vi "Test and Get Data.vi"(5 "Point #":i32, 6 "Eng Units?":bool, 7 "error in (no error)":errorcluster, 8 "Instrument Info":T1={"Instrument"="Instrument", "ID Test String"="", "Terminator Character"="", "wait (mS)"=0, "Wait For SRQ"=FALSE}, 9 "Command String":string, 10 "VISA Sesson":refnum<visa-resource-name>) -> (0 "Error Out":errorcluster, 1 "Measurement":dbl[](array[numeric]), 2 "String Response":string, 3 "dup VISA session":refnum<visa-resource-name>, 4 "Stop":bool)   [LabVIEW 2019]
doc: "This VI reads tests for presence of an instrument on the GPIB bus for an index <0. It also gets one reading from an instrument. If no reading is obtained a single zero is returned.\nScott Hannahs, <sth@magnet.fsu.edu> NHMFL-FSU, May 2003"
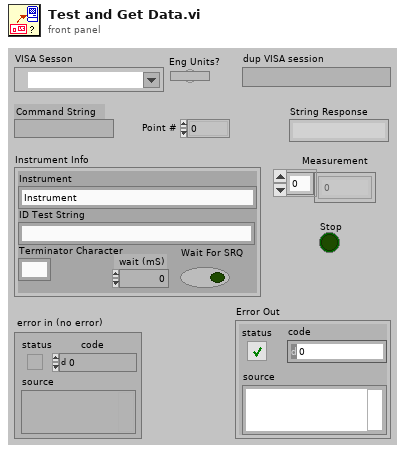
[diagram p1: front panel]
types:
  T1 = cluster{"Instrument":string, "ID Test String":string, "Terminator Character":string, "wait (mS)":u32, "Wait For SRQ":bool}
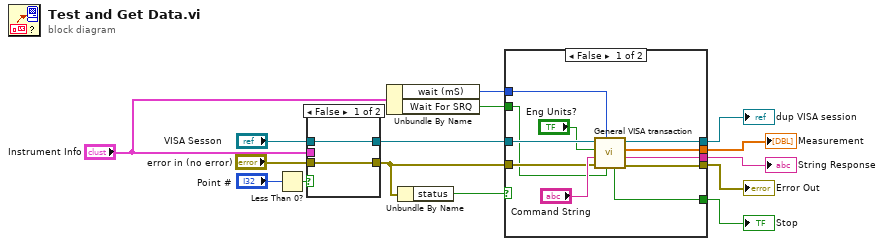
[diagram p0: block diagram]
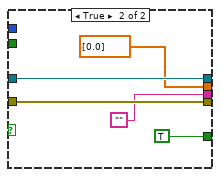
[diagram p2: hidden frame]
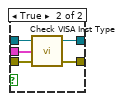
[diagram p3: hidden frame]
diagram:
  n1 = Less Than 0?(x="Point #") -> (x < 0?=w3:bool)
  n2 = case shown="False" w3 {
    tunnel: "Instrument Info" -> [_ w22]
    tunnel: "VISA Sesson" -> [w17 w21]
    tunnel: [w16 w20] -> w7
    tunnel: [w17 w19] -> w6
    tunnel: "error in (no error)" -> [w16 w18]
    frame False {
    }
    frame True {
      n3 = call "Check VISA Inst Type.vi"("Error In"=w18, "Check Parameters"=w22, "VISA session"=w21) -> ("Error Out"=w20:errorcluster, "dup VISA session"=w19:refnum<visa-resource-name>)  [unwired: 1 out]
    }
  }
  n4 = Unbundle By Name("Instrument Info") -> ("wait (mS)"=w10:u32, "Wait For SRQ"=w11:bool)
  n5 = Unbundle By Name(w7) -> ("status"=w5:bool)
  n6 = case shown="False" w5 {
    tunnel: w6 -> [w33 w38]
    tunnel: [w32 w38] -> w12
    tunnel: [w27 w37] -> w8
    tunnel: w7 -> [w25 w37]
    tunnel: [w26 TRUE] -> w9
    tunnel: [w31 dbl[] [0.0] ("Measurement")] -> w14
    tunnel: [w30 ""] -> w15
    tunnel: w10 -> [w23 _]
    tunnel: w11 -> [w24 _]
    frame False {
      n7 = call "General VISA transaction.vi"("Wait For SRQ"=w24, "Wait (mS)"=w23, "error in (no error)"=w25, "Command String"="Command String", "Eng Units?"="Eng Units?", "VISA Session"=w33) -> ("error out"=w27:errorcluster, "String Resonse"=w30:string, "Measurement"=w31:dbl[], "dup VISA Session"=w32:refnum<visa-resource-name>, "Stop"=w26:bool)  [unwired: 1 out]
    }
    frame True {
    }
  }
  "dup VISA session" <- w12
  "Error Out" <- w8
  "Stop" <- w9
  "Measurement" <- w14
  "String Response" <- w15
